vi "正面结果分析.vi"(11 "元素":T2 {"Correlation Score" format="%.2f"; "Target Template Curve Score" format="%.2f"; "Template Target Curve Score" format="%.2f"; "Bounding Box"."y" format="%.2f"; "Bounding Box"."x" format="%.2f"; "Position"."y" format="%.2f"; "Position"."x" format="%.2f"; "Score" format="%.2f"; "Scale" format="%.2f"; "Angle" format="%.2f"; "Occlusion %" format="%.2f"}) -> (0 "添加的数组 2":string[](array[string]), 2 "Angle":sgl, 3 "添加的数组":T1(array[cluster]))   [LabVIEW 2017]
uses:
  <vilib>/vision/Pattern Matching.llb/IMAQ GM Match Report.ctl
  Global System.vi
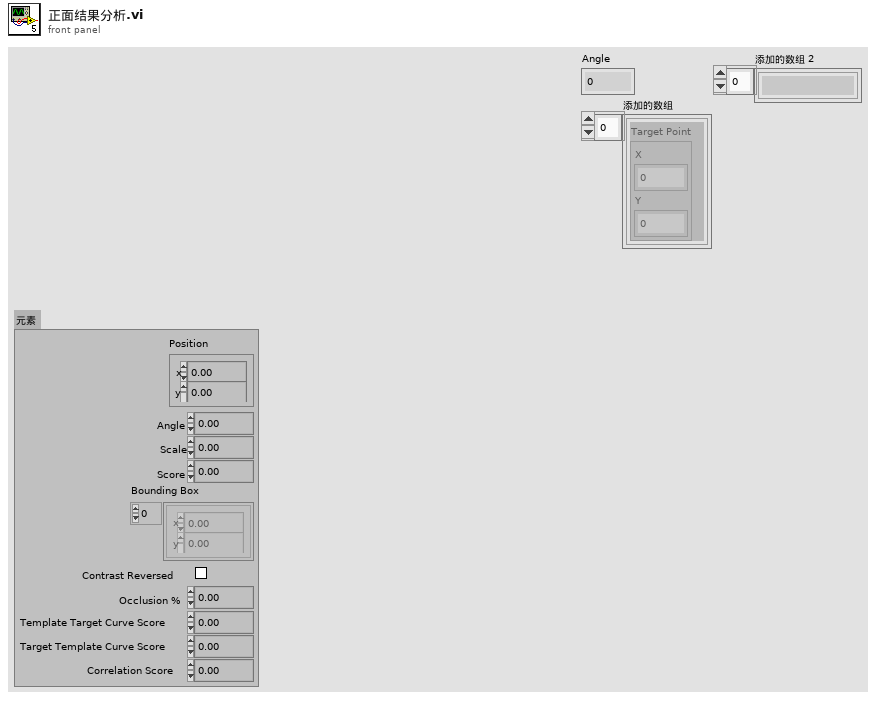
[diagram p1: front panel]
types:
  T1 = cluster{"Target Point":cluster{"X":dbl, "Y":dbl}}[]
  T2 = typedef "IMAQ GM Match Report.ctl" = cluster{"Position":cluster{"x":sgl, "y":sgl}, "Angle":sgl, "Scale":sgl, "Score":sgl, "Bounding Box":cluster{"x":sgl, "y":sgl}[], "Contrast Reversed":bool, "Occlusion %":sgl, "Template Target Curve Score":sgl, "Target Template Curve Score":sgl, "Correlation Score":sgl}
  T3 = cluster{"Target Point":cluster{"X":dbl, "Y":dbl}}
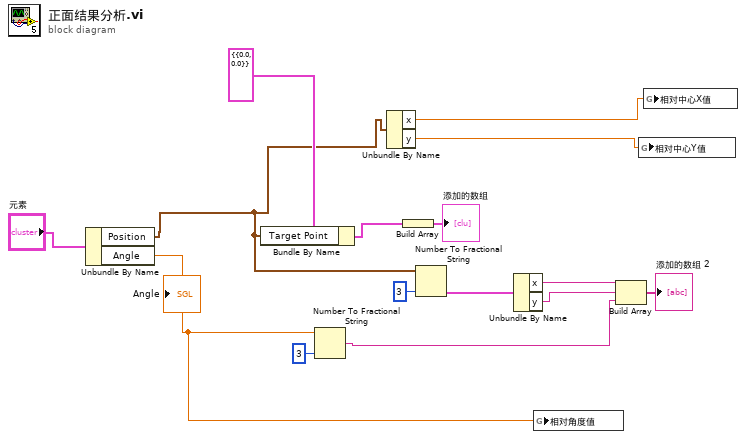
[diagram p0: block diagram]
diagram:
  n1 = Unbundle By Name("元素") -> ("Position"=w4:cluster{"x":sgl, "y":sgl}, "Angle"=w1:sgl)
  "Angle" <- w1
  n2 = Bundle By Name(cluster=T3 {"Target Point"={"X"=0.0, "Y"=0.0}} ("Cluster"), "Target Point"=w4) -> (w12:T3)
  n3 = Number To Fractional String(number=w1, precision (6)=i16 3 ("精度(6)")) -> (F-format string=w7:string)  [unwired: 2 in]
  n4 = Unbundle By Name(w4) -> ("x"=w3:sgl, "y"=w2:sgl)
  n5 = Build Array(w12) -> (→"添加的数组":T1)
  n6 = Number To Fractional String(number=w4, precision (6)=i16 3 ("精度(6)")) -> (F-format string=w10:cluster{"x":string, "y":string})  [unwired: 2 in]
  n7 = Unbundle By Name(w10) -> ("x"=w9:string, "y"=w8:string)
  n8 = global write "Global System.vi" "相对角度值"(w1) -> ()
  n9 = Build Array(w9, w8, w7) -> (→"添加的数组 2":string[])
  n10 = global write "Global System.vi" "相对中心Y值"(w2) -> ()
  n11 = global write "Global System.vi" "相对中心X值"(w3) -> ()
